vi "Trial Start flag cleanup.vi"   [LabVIEW 2013]
uses:
  Typedefs/HW config states enum.ctl
  typedefs/Functions enum.ctl
types:
  T1 = typedef "HW config states enum.ctl" = enum16{"Load from file", "Save to file", "Write all", "Read all", "Write XY stage settings", "Write DAQ FPGA settings", "Write Control FPGA settings", "Write Phys Channels", "Clear", "Compare from file"}
  T2 = typedef "Sys Configuration.ctl" = cluster{"XY Stage":T3, "DAQ FPGA":T4, "Control system":T8, "Encoder":T9, "DAQmx Chan":T10, "Computer MAC address":string, "Cam VidRec":T11, "Externalise Triggers":bool, "Laser wavelength (nm)":dbl}
  T3 = typedef "XY Stage config cluster.ctl" = cluster{"COM port":refnum<visa-resource-name>, "XY stage available":bool}
  T4 = typedef "DAQ FPGA config cluster.ctl" = cluster{"Ref":T5, "Target":T6, "Clock Freq (MHz) ":dbl, "input card type":T7, "Samples Wait after Trigger":u16, "AOD fill":u16, "StartupDelay":i32, "Slip Cycle (clock cycles)":u32, "Add Cycle":bool}
  T5 = typedef "FPGA Ref.ctl" = refnum<k20>
  T6 = typedef "nirio_resource_hc.ctl" = tag
  T7 = typedef "FPGA input type AC-DC.ctl" = enum16{"AC Card", "DC Card"}
  T8 = typedef "CTRL system config cluster.ctl" = cluster{"Ethernet opened":bool, "Ethernet Port":u32, "Ctrl FPGA available":bool, "Ctrl FPGA Clock (MHz)":dbl, "Ctrl system MAC address":string, "Control system.Network adapter name":string, "AOD 1 Amplitude":i16, "AOD 2 Amplitude":i16, "AOD 3 Amplitude":i16, "AOD 4 Amplitude":i16, "Data Time Interval (ns)":dbl, "T0 (ns)":dbl, "Ta (ns)":dbl}
  T9 = typedef "Encoder config cluster.ctl" = cluster{"IP address":string, "Port":u16, "Encoder available":bool, "Wheel radius (cm)":dbl}
  T10 = typedef "DAQmx physical channels cluster.ctl" = cluster{"Pockels AO":tag, "Hard shutter AO":tag, "PMT AOs":tag, "Power meter AI":tag}
  T11 = typedef "Cam VidRec HW config setup cluster.ctl" = cluster{"DO flag-Video record":tag, "DO flag-Trial start":tag, "VidRec available":bool}
  T12 = typedef "Functions enum.ctl" = enum16{"Create", "Start", "Write", "Stop", "Clear"}
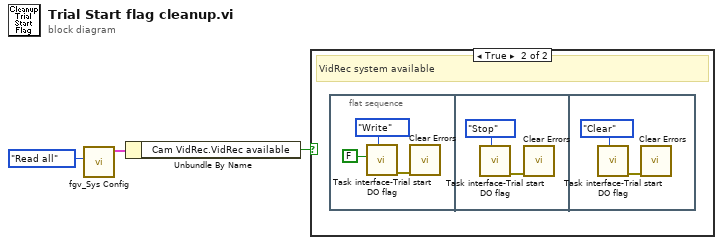
[diagram p0: block diagram]
diagram:
  n1 = call "fgv_Sys Config.vi"("Function"=HW_config_states_enum."Read all") -> ("System Config out"=w2:T2)  [unwired: 9 in, 1 out]
  n2 = Unbundle By Name(w2) -> ("Cam VidRec.VidRec available"=w1:bool)
  n3 = case shown="True" w1 {
    frame False {
      # "VidRec system unavailable"
    }
    frame True {
      # "VidRec system available"
      n4 = flat-sequence {
        frame #0 {
          n5 = call "Task interface-Trial start DO flag.vi"("Function"=Functions_enum."Write", "DO value"=FALSE) -> ("error out"=w4:errorcluster)  [unwired: 9 in]
          n6 = call <vilib>:"Clear Errors.vi"("error in (no error)"=w4) -> ()  [unwired: 6 in, 1 out]
        }
        frame #1 {
          n7 = call "Task interface-Trial start DO flag.vi"("Function"=Functions_enum."Stop") -> ("error out"=w7:errorcluster)  [unwired: 10 in]
          n8 = call <vilib>:"Clear Errors.vi"("error in (no error)"=w7) -> ()  [unwired: 6 in, 1 out]
        }
        frame #2 {
          n9 = call "Task interface-Trial start DO flag.vi"("Function"=Functions_enum."Clear") -> ("error out"=w9:errorcluster)  [unwired: 10 in]
          n10 = call <vilib>:"Clear Errors.vi"("error in (no error)"=w9) -> ()  [unwired: 6 in, 1 out]
        }
      }
    }
  }
